vi "TP_GV_UI_Ref.vi"() -> ()   [LabVIEW 2012]
uses:
  controls/TP_UI Ref.ctl
panel:
  out "output cluster":T1
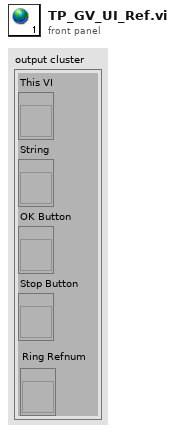
[diagram p1: front panel]
types:
  T1 = typedef "TP_UI Ref.ctl" = cluster{"This VI":refnum<vi>, "String":refnum<vi>, "OK Button":refnum<vi>, "Stop Button":refnum<vi>, "Ring Refnum":refnum<vi>}
diagram:
